vi "Update Plot.vi"(4 "Good fit?":dbl[](array[numeric]) format="%#_4p", 6 "Peak Plot":cluster{"Ramp Pattern":dbl[], "X":dbl[]}[](array[cluster]), 8 "error in (no error)":errorcluster, 9 "Plots":cluster{"X":dbl[], "Array":dbl[]}[](array[cluster]), 10 "Best fit results":dbl[][](array[numeric]) format="%#_4p", 11 "Resonance Detector in":refnum<class "Resonance Detector.lvclass">) -> (0 "error out":errorcluster, 3 "Resonance Detector out":refnum<class "Resonance Detector.lvclass">)   [LabVIEW 2020, in "Resonance Detector.lvclass"]
uses:
  Resonance Detector.lvclass
  Resonance Detector.lvclass/Resonance Detector.ctl
panel:
  # "F0         dF     Ampl   Phase   Xbgrd   Ybgrd"
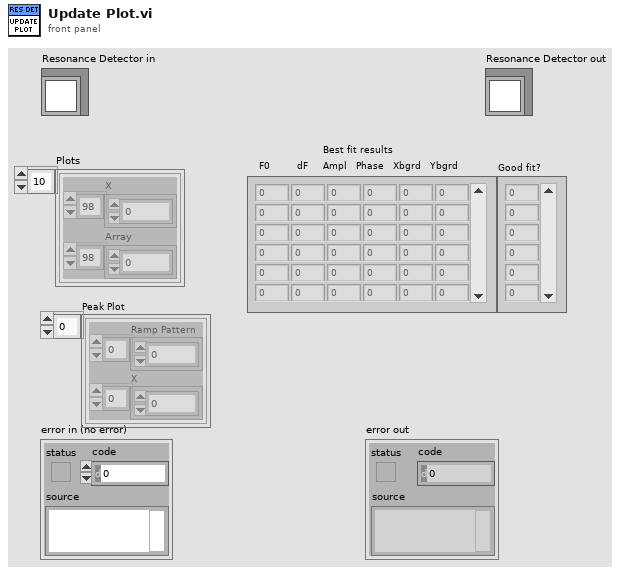
[diagram p1: front panel]
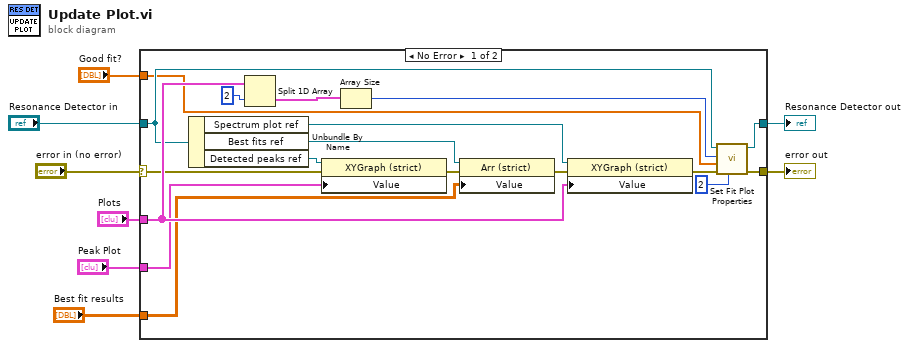
[diagram p0: block diagram]
diagram:
  n1 = case shown="No Error" "error in (no error)" {
    selector: "error in (no error)" -> [w18 w28]
    tunnel: [w12 w28] -> w7
    tunnel: [w14 w27] -> w5
    tunnel: "Resonance Detector in" -> [w15 w27]
    tunnel: "Plots" -> [w19 _]
    tunnel: "Best fit results" -> [w17 _]
    tunnel: "Peak Plot" -> [w16 _]
    tunnel: "Good fit?" -> [w11 _]
    frame No Error {
      n2 = Unbundle By Name(w15) -> ("Spectrum plot ref"=w25:refnum<vi>, "Best fits ref"=w21:refnum<vi>, "Detected peaks ref"=w20:refnum<vi>)
      n3 = Split 1D Array(array=w19, index=2) -> (second subarray=w24:cluster{"X":dbl[], "Array":dbl[]}[])  [unwired: 1 out]
      n4 = property class="XYGraph (strict)"(reference=w20, error in=w18, "Value"=w16) -> (error out=w22:errorcluster)  [unwired: 1 out]
      n5 = Array Size(array=w24) -> (size(s)=w10:i32)
      n6 = property class="Arr (strict)"(reference=w21, error in=w22, "Value"=w17) -> (error out=w26:errorcluster)  [unwired: 1 out]
      n7 = property class="XYGraph (strict)"(reference=w25, error in=w26, "Value"=w19) -> (error out=w13:errorcluster)  [unwired: 1 out]
      n8 = call-dynamic "Set Fit Plot Properties.vi"("Fit array start"=2, "error in (no error)"=w13, "Good fit?"=w11, "Fit array size"=w10, "Resonance Detector in"=w15) -> ("error out"=w12:errorcluster, "Resonance Detector out"=w14:refnum<class "Resonance Detector.lvclass">)  [unwired: 5 in]
    }
    frame Error {
    }
  }
  "error out" <- w7
  "Resonance Detector out" <- w5
